vi "UI.vi"() -> ()   [LabVIEW 2024]
uses:
  Module/AddModuleParams.ctl
  Helper/AddHelper.lvlib
  Event/AddNewEvent.lvlib
  Module/AddNewModule.lvlib
panel:
  in  "Module":u16(ring) items=["ModuleManager", "ErrorHandler", "Header", "Shell", "Layout", "TitleBar", "UIManager", "NewTemplate", "TemplateModule"]
  in  "Add Button":bool
  in  "Tab Control":T1(tab)
  in  "Request Name":string caption="Name"
  in  "Broadcast Name":string caption="Name"
  in  "Helper Name":string caption="Name"
  in  "Module Tester VI":path=path "C:/DevOps/CORTEX/JQMH/ModuleTemplates/NewTemplateModule/NewTemplate.Tester.vi"
  in  "Template Module":path=path "C:/DevOps/CORTEX/JQMH/ModuleTemplates/NewTemplateModule/NewTemplate.lvclass"
  in  "Save Folder":path=path "C:/DevOps/CORTEX/JQMH/ModuleTemplates"
  in  "New Module Name":string caption="Name"
  # "Prove out UI for the concept of VI scripting a module"
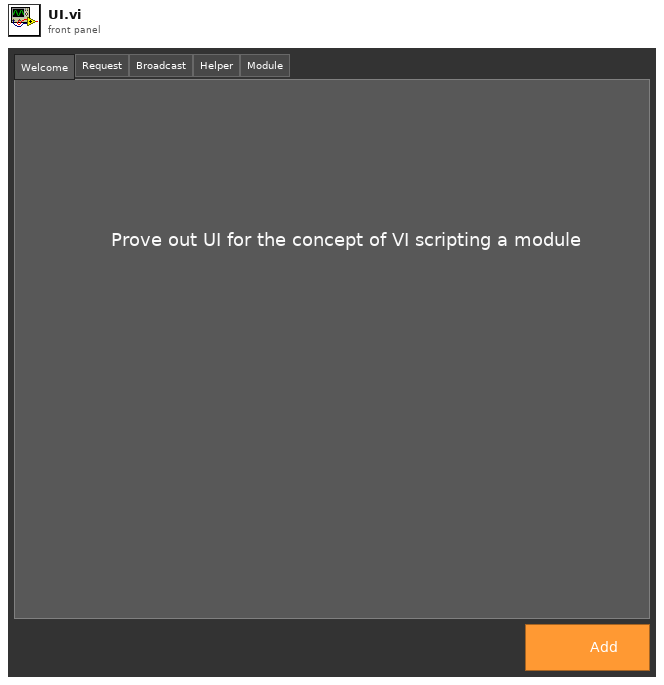
[diagram p1: front panel]
types:
  T1 = enum32{"Welcome", "Request", "Broadcast", "Helper", "Module"}
  T2 = typedef "AddNewModule.lvlib/AddModuleParams.ctl" = cluster{"Template Class Path":path, "Tester Path":path, "Name":string}
  T3 = enum32{"Invalid", "Standard", "Closed", "Hidden", "Minimized", "Maximized"}
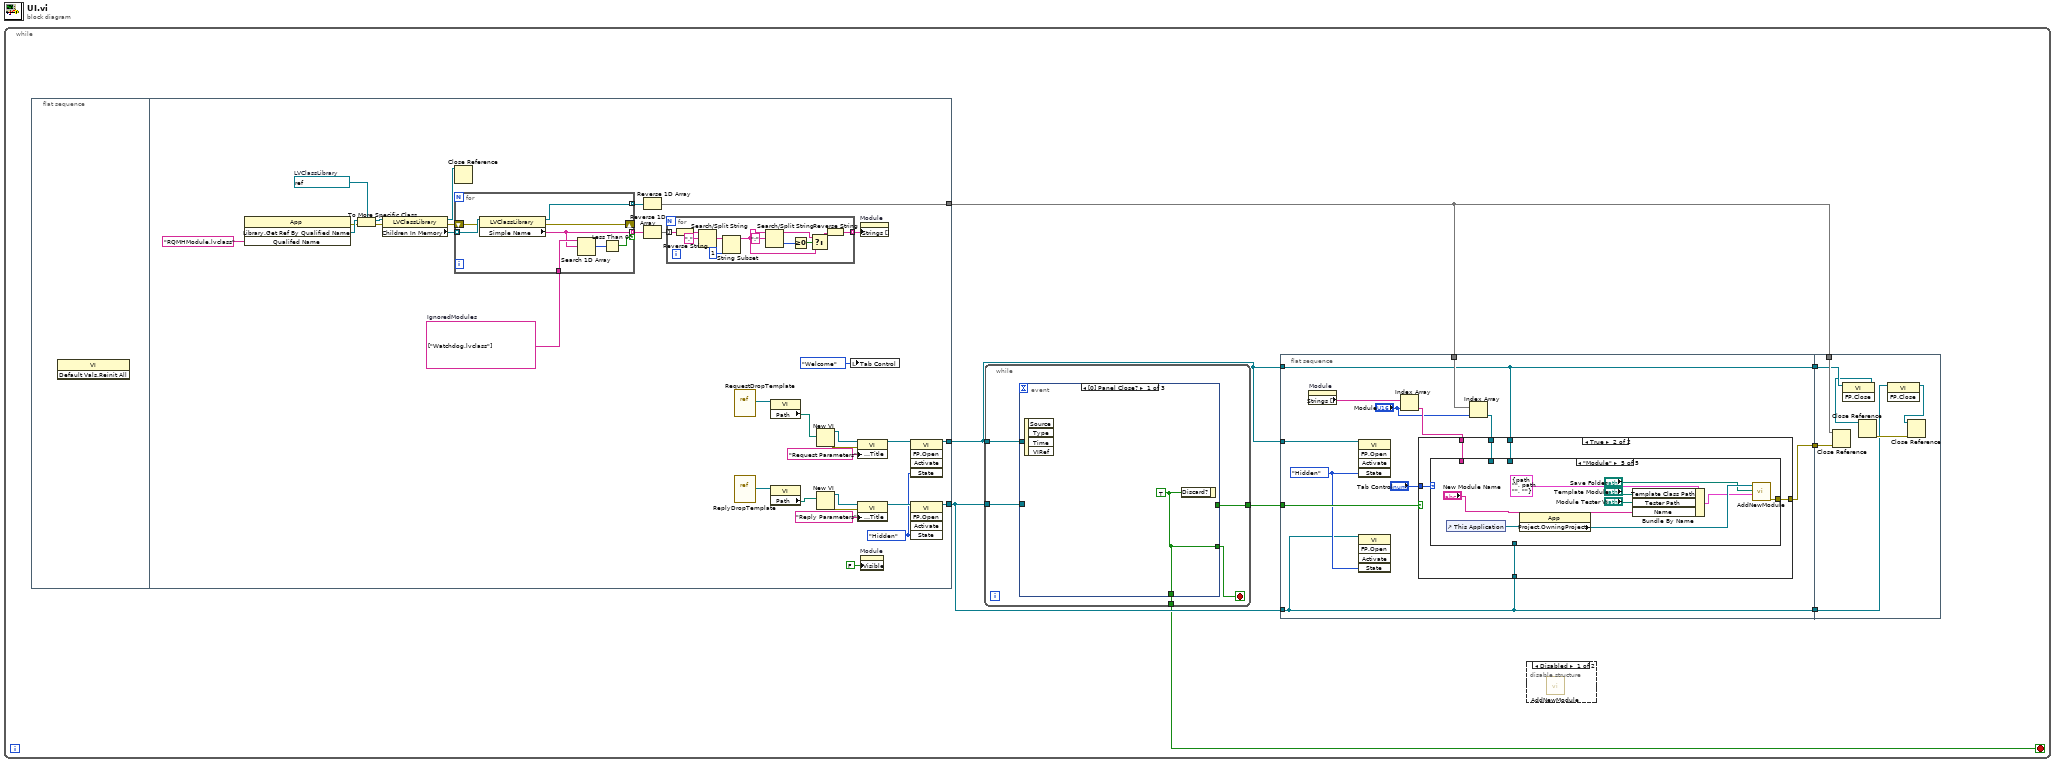
[diagram p0: block diagram]
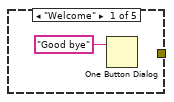
[diagram p4: hidden frame]
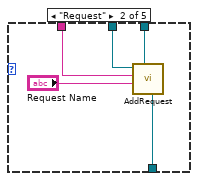
[diagram p5: hidden frame]
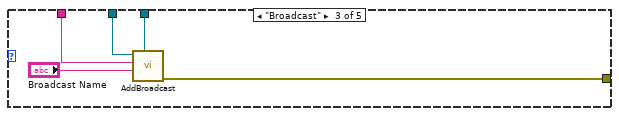
[diagram p6: hidden frame]
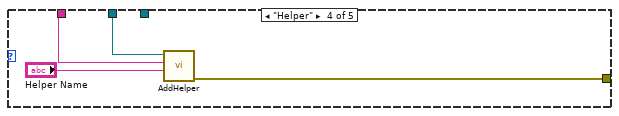
[diagram p7: hidden frame]
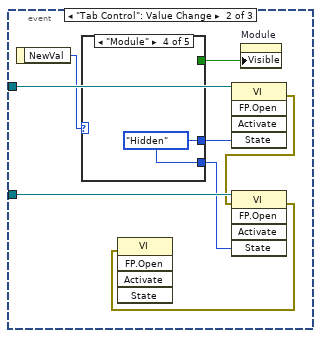
[diagram p8: hidden frame]
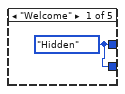
[diagram p9: hidden frame]
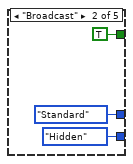
[diagram p10: hidden frame]
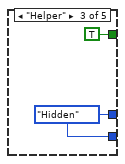
[diagram p11: hidden frame]
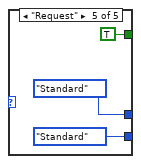
[diagram p12: hidden frame]
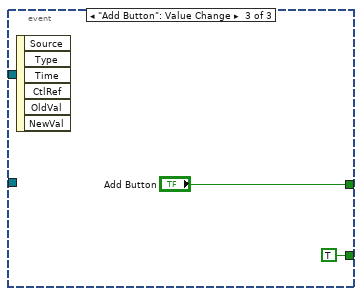
[diagram p13: hidden frame]
diagram:
  n1 = while {
    stop <- w1 stop-if-true
    n2 = flat-sequence {
      tunnel: [w26] -> w4
      tunnel: [w16] -> w3
      tunnel: [w14] -> w2
      frame #0 {
        n3 = invoke class="VI" method="Default Vals.Reinit All"() -> ()  [unwired: 3 in, 3 out]
      }
      frame #1 {
        w9 = string[] ["Watchdog.lvclass"]  # IgnoredModules
        w23 = refnum<vi> refnum  # LVClassLibrary
        w31 = T3."Hidden" ("State")
        n4 = invoke class="App" method="Library.Get Ref By Qualified Name"("Qualifed Name"="RQMHModule.lvclass" ("class name 2")) -> (error out=w24:errorcluster, "Library.Get Ref By Qualified Name"=w25:refnum<vi>)  [unwired: 3 in, 2 out]
        n5 = To More Specific Class(target class=w23, reference=w25, error in=w24) -> (specific class reference=w10:refnum<vi>, error out=w22:errorcluster)
        n6 = property class="LVClassLibrary"(reference=w10, error in=w22) -> (reference out=w19:refnum<vi>, error out=w20:errorcluster, "Children In Memory"=w21:refnum<vi>[])
        n7 = Close Reference(reference=w19) -> ()  [unwired: 1 in, 1 out]
        n8 = for {
          tunnel: w21 -> [w60] mode=indexing
          shift-right: [w58] -> _
          shift-left: w20 -> [w59]
          tunnel: [w55] -> w18 mode=indexing if=w53
          tunnel: [w57] -> w15 mode=indexing
          tunnel: w9 -> [w56]
          n9 = property class="LVClassLibrary"(reference=w60, error in=w59) -> (reference out=w57:refnum<vi>, error out=w58:errorcluster, "Simple Name"=w55:string)
          n10 = Search 1D Array(1D array=w56, element=w55) -> (index of element=w54:i32)  [unwired: 1 in]
          n11 = Less Than 0?(x=w54) -> (x < 0?=w53:bool)
        }
        n12 = Reverse 1D Array(array=w15) -> (reversed array=w14:refnum<vi>[])
        n13 = Reverse 1D Array(array=w18) -> (reversed array=w12:string[])
        n14 = for {
          tunnel: [w44] -> w13 mode=indexing
          tunnel: w12 -> [w52] mode=indexing
          n15 = Reverse String(1:w52) -> (0:w51:string)
          n16 = Search/Split String(string=w51, search string/char (-)="." ("match + rest of string")) -> (match + rest of string=w43:string)  [unwired: 1 in, 2 out]
          n17 = String Subset(string=w43, offset (0)=1) -> (substring=w42:string)  [unwired: 1 in]
          n18 = Search/Split String(string=w42, search string/char (-)=":") -> (substring before match=w46:string, offset of match=w48:i32)  [unwired: 1 in, 1 out]
          n19 = Greater Or Equal To 0?(x=w48) -> (x >= 0?=w47:bool)
          n20 = Select(t=w46, s=w47, f=w42) -> (s? t:f=w45:string)
          n21 = Reverse String(1:w45) -> (0:w44:string)
        }
        n22 = vi-ref "RequestDropTemplate.vi"() -> (w30:refnum<vi>)
        n23 = vi-ref "ReplyDropTemplate.vi"() -> (w28:refnum<vi>)
        n24 = property class="VI"(reference=w30) -> ("Path"=w29:path)  [unwired: 1 in, 2 out]
        n25 = property class="VI"(reference=w28) -> ("Path"=w27:path)  [unwired: 1 in, 2 out]
        n26 = New VI(10:w29) -> (0:w40:errorcluster, 3:w39:refnum<vi>)  [unwired: 6 in]
        n27 = New VI(10:w27) -> (0:w35:errorcluster, 3:w36:refnum<vi>)  [unwired: 6 in]
        n28 = local write "Tab Control"(enum32{"Welcome", "Request", "Broadcast"}."Welcome" ("Tab Control")) -> ()
        n29 = property class="VI"(reference=w39, error in=w40, "Front Panel.Title"="Request Parameters" ("Front Panel Window:Title")) -> (reference out=w32:refnum<vi>)  [unwired: 1 out]
        n30 = property class="VI"(reference=w36, error in=w35, "Front Panel.Title"="Reply Parameters" ("Front Panel Window:Title")) -> (reference out=w33:refnum<vi>)  [unwired: 1 out]
        n31 = property on="Module" class="Ring (strict)"("Strings []"=w13) -> ()  [unwired: 2 in, 2 out]
        n32 = property on="Module" class="Ring (strict)"("Visible"=FALSE) -> ()  [unwired: 2 in, 2 out]
        n33 = invoke class="VI" method="FP.Open"(reference=w32, "State"=w31) -> (reference out=w16:refnum<vi>)  [unwired: 3 in, 4 out]
        n34 = invoke class="VI" method="FP.Open"(reference=w33, "State"=w31) -> (reference out=w26:refnum<vi>)  [unwired: 3 in, 4 out]
      }
    }
    n35 = while {
      tunnel: w4 -> [w112]
      tunnel: w3 -> [w113]
      tunnel: [w111] -> w5
      tunnel: [w110] -> w1
      stop <- w114 stop-if-true
      n36 = event shown="[0] Panel Close?" {
        selector: _ -> [_ _ _]
        dyn-events: _ -> [_ _ _]
        timeout: _ -> [_ _ _]
        tunnel: [w115 _ TRUE] -> w114
        tunnel: w113 -> [_ w123 _]
        tunnel: w112 -> [_ w122 _]
        tunnel: [_ _ "Add Button"] -> w111
        tunnel: [w115 _ _] -> w110
        event Panel Close? {
          w115 = TRUE
          n37 = event-data() -> ()  [unwired: 1 in, 4 out]
          n38 = event-data("Discard?"=w115) -> ()  [unwired: 1 in, 1 out]
        }
        event "Tab Control": Value Change {
          n39 = event-data() -> ("NewVal"=w121:T1)  [unwired: 1 in]
          n40 = case shown="\"Module\"" w121 {
            tunnel: [w124 T3."Standard" ("State") w129 w130 T3."Standard" ("State")] -> w120
            tunnel: [w124 T3."Hidden" ("State") w129 w130 T3."Standard" ("State")] -> w119
            tunnel: [_ TRUE ("Visible") TRUE ("Visible") _ TRUE ("Visible")] -> w118
            frame "Welcome" {
              w124 = T3."Hidden" ("State")
            }
            frame "Broadcast" {
            }
            frame "Helper" {
              w129 = T3."Hidden" ("State")
            }
            frame "Module" {
              w130 = T3."Hidden" ("State")
            }
            frame "Request" {
            }
          }
          n41 = invoke class="VI" method="FP.Open"(reference=w123, "State"=w120) -> (error out=w116:errorcluster)  [unwired: 3 in, 4 out]
          n42 = invoke class="VI" method="FP.Open"(reference=w122, error in=w116, "State"=w119) -> (error out=w117:errorcluster)  [unwired: 2 in, 4 out]
          n43 = invoke class="VI" method="FP.Open"(error in=w117) -> ()  [unwired: 4 in, 5 out]
          n44 = property on="Module" class="Ring (strict)"("Visible"=w118) -> ()  [unwired: 2 in, 2 out]
        }
        event "Add Button": Value Change {
          n45 = event-data() -> ()  [unwired: 1 in, 6 out]
        }
      }
    }
    n46 = flat-sequence {
      tunnel: w5 -> [w72]
      tunnel: w3 -> [w69]
      tunnel: w4 -> [w62]
      tunnel: w3 -> [w61]
      tunnel: w2 -> [w64]
      tunnel: [w63] -> w8
      tunnel: [w62] -> w7
      tunnel: [w61] -> w6
      tunnel: w8 -> [w108]
      tunnel: w2 -> [w107]
      tunnel: w7 -> [w106]
      tunnel: w6 -> [w105]
      frame #0 {
        w70 = T3."Hidden" ("State")
        n47 = property on="Module" class="Ring (strict)"() -> ("Strings []"=w68:string[])  [unwired: 2 in, 2 out]
        n48 = invoke class="VI" method="FP.Open"(reference=w69, "State"=w70) -> ()  [unwired: 3 in, 5 out]
        n49 = invoke class="VI" method="FP.Open"(reference=w62, "State"=w70) -> ()  [unwired: 3 in, 5 out]
        n50 = Index Array(array=w68, index="Module") -> (element=w67:string)
        n51 = Index Array(array=w64, index="Module") -> (element=w65:refnum<vi>)
        n52 = case shown="True" w72 {
          tunnel: "Tab Control" -> [_ w78]
          tunnel: w67 -> [_ w77]
          tunnel: w61 -> [_ w76]
          tunnel: w62 -> [_ w75]
          tunnel: w65 -> [_ w74]
          tunnel: [_ w73] -> w63
          frame False {
          }
          frame True {
            n53 = case shown="\"Module\"" w78 {
              tunnel: w77 -> [_ w81 w87 w91 _]
              tunnel: w76 -> [_ w84 w89 _ _]
              tunnel: w75 -> [_ w83 _ _ _]
              tunnel: w74 -> [_ w80 w88 w92 _]
              tunnel: [_ _ w85 w93 w102] -> w73
              frame "Welcome" {
                n54 = One Button Dialog(message="Good bye") -> ()  [unwired: 1 in, 1 out]
              }
              frame "Request" {
                n55 = call "AddRequest.vi"("Reply Params Source"=w83, "Request Params Source"=w84, "Request Name"="Request Name", "Module Name"=w81, "Module Ref"=w80) -> ()  [unwired: 7 in]
              }
              frame "Broadcast" {
                n56 = call "AddBroadcast.vi"("Broadcast Params"=w89, "Broadcast Name"="Broadcast Name", "Module Name"=w87, "Module Ref"=w88) -> ("error out"=w85:errorcluster)  [unwired: 7 in]
              }
              frame "Helper" {
                n57 = call "AddHelper.vi"("Helper Name"="Helper Name", "Module Name"=w91, "Module Ref"=w92) -> ("error out"=w93:errorcluster)  [unwired: 8 in]
              }
              frame "Module" {
                n58 = control-ref of="This Application"() -> (w101:refnum<vi>)
                n59 = property class="App"(reference=w101) -> ("Project.OwningProject"=w100:refnum<vi>)  [unwired: 1 in, 2 out]
                n60 = Bundle By Name(cluster=T2 {"Template Class Path"=path "", "Tester Path"=path "", "Name"=""} ("ModuleParams"), "Template Class Path"="Template Module", "Tester Path"="Module Tester VI", "Name"="New Module Name") -> (w98:T2)
                n61 = call "AddNewModule.vi"("ModuleParams"=w98, "Save Folder"="Save Folder", "Project in"=w100) -> ("error out"=w102:errorcluster)  [unwired: 7 in, 1 out]
              }
            }
          }
        }
      }
      frame #1 {
        n62 = Close Reference(reference=w107, error in (no error)=w108) -> ()  [unwired: 1 out]
        n63 = invoke class="VI" method="FP.Close"(reference=w105) -> (reference out=w104:refnum<vi>)  [unwired: 2 in, 2 out]
        n64 = Close Reference(reference=w104) -> (error out=w109:errorcluster)  [unwired: 1 in]
        n65 = invoke class="VI" method="FP.Close"(reference=w106) -> (reference out=w103:refnum<vi>)  [unwired: 2 in, 2 out]
        n66 = Close Reference(reference=w103, error in (no error)=w109) -> ()  [unwired: 1 out]
      }
    }
    n67 = disable-structure shown="Disabled" {
      frame Disabled {
        n68 = call "AddNewModule.vi"() -> ()  [unwired: 10 in, 2 out]
      }
      frame Enabled {
      }
    }
  }
